vi "init.vi"(8 "error in (no error)":errorcluster, 10 "Scan Settings":T1={"Amplitude Scan Settings"={"Start Value"=1.0, "Stop Value"=1.0, "Steps"=2}, "Rate Scan Settings"=[], "Sample Count"=0, "Iterations"=0.0, "Amplitude"=0.0, "Offset"=0.0, "Frequency"=0.0, "Waveform"=enum."Sine", "F1"=0.0, "F2"=0.0, "Duty Cycle"=0.0, "ILC Rate"=0.0, "Operator"="", "Scan Name"="", "Notes"="", "Ramp Time"=0.0, "Hold Time"=0.0, "Settling Time"=0.0} {"Amplitude Scan Settings"."Stop Value" format="%.3f"; "Amplitude Scan Settings"."Start Value" format="%.3f"}, 11 "WaveformGenerator in":refnum<class "WaveformGenerator.lvclass">) -> (0 "error out":errorcluster, 3 "WaveformGenerator out":refnum<class "WaveformGenerator.lvclass">)   [LabVIEW 2015, in "WaveformGenerator.lvclass"]
uses:
  WaveformGenerator.lvclass
  Typedefs/Scan Settings.ctl
  Typedefs/Test Values.ctl
  <userlib>/Common/ILC/Configuration/Scan Rates.ctl
  Typedefs/Waveform.ctl
  WaveformGenerator.lvclass/WaveformGenerator.ctl
  Typedefs/FAMTTypedefs.lvlib
  <userlib>/Common/ILC/Configuration/ILCConfiguration.lvlib
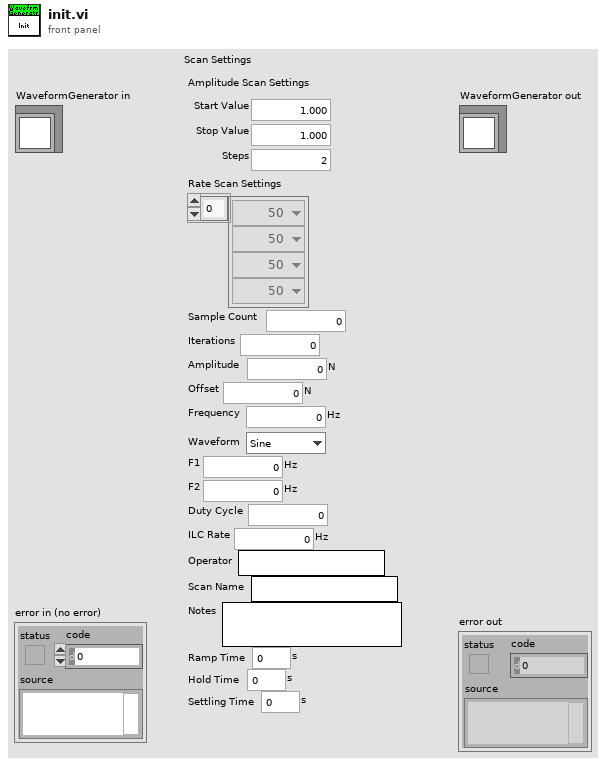
[diagram p1: front panel]
types:
  T1 = typedef "FAMTTypedefs.lvlib/Scan Settings.ctl" = cluster{"Amplitude Scan Settings":T2, "Rate Scan Settings":T3[], "Sample Count":u32, "Iterations":dbl, "Amplitude":dbl[unit], "Offset":dbl[unit], "Frequency":dbl[unit], "Waveform":T4, "F1":dbl[unit], "F2":dbl[unit], "Duty Cycle":dbl, "ILC Rate":dbl[unit], "Operator":string, "Scan Name":string, "Notes":string, "Ramp Time":dbl[unit], "Hold Time":dbl[unit], "Settling Time":dbl[unit]}
  T2 = typedef "FAMTTypedefs.lvlib/Test Values.ctl" = cluster{"Start Value":dbl, "Stop Value":dbl, "Steps":u16}
  T3 = typedef "ILCCommon.lvlib/ILCConfiguration.lvlib/Scan Rates.ctl" = enum16{"50", "60", "100", "120", "200", "240", "300", "400", "480", "600", "1200", "2400", "4800"}
  T4 = typedef "FAMTTypedefs.lvlib/Waveform.ctl" = enum16{"Sine", "Triangle", "Square", "Sawtooth", "Chirp", "Gaussian", "Trapezoid"}
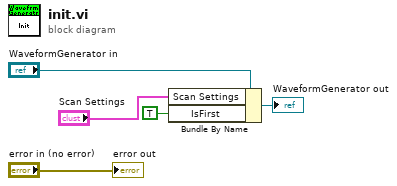
[diagram p0: block diagram]
diagram:
  n1 = Bundle By Name(cluster="WaveformGenerator in", "Scan Settings"="Scan Settings", "IsFirst"=TRUE) -> (→"WaveformGenerator out":refnum<class "WaveformGenerator.lvclass">)
  "error out" <- "error in (no error)"
